vi "Subvi_Online_For_Offline_Analysis_For_Checking_LDAMatrix_w_weight.vi"(0 "rate":dbl=500.0 caption="Rate" format="%0.2f", 1 "samples per channel":i32=25, 5 "Brain_data_source":dbl[][](array[numeric]) caption="EEG_Raw_Data" format="%0.3f", 7 "Target_Flash_Order":i64[][](array[numeric]), 8 "Value":T1, 9 "사용할 Parameter 갯수":i32=2, 10 "Weight":dbl[](array[numeric]), 11 "Path":path, 14 "Number":string, 16 "Matrix":T1, 17 "Channel selection":bool[](array[boolean])) -> (13 "Array":dbl[](array[numeric]), 15 "자극별 ERP 발생여부":i16[](array[numeric]), 20 "output-0~8":i32, 24 "ERP_all":dbl[][](array[numeric]), 25 "자극별 ERP 발생 총 횟수":i16[](array[numeric]))   [LabVIEW 2014]
uses:
  <vilib>/Analysis/Matrix/Datatypes/RealMatrix.ctl
  <vilib>/Analysis/3filter.llb/Filter Passband Type.ctl
  <vilib>/Analysis/baseanly.llb/Real A x B.vi
  <vilib>/Analysis/baseanly.llb/Mean (DBL).vi
  <vilib>/Analysis/3filter.llb/Butterworth Filter (DBL).vi
  <vilib>/Analysis/Matrix/Numeric/Conversions/Array To Matrix - RA.vi
  <vilib>/Analysis/Matrix/Numeric/Conversions/Array To Matrix - RA2.vi
  <vilib>/Analysis/Matrix/Numeric/Conversions/Matrix To Array - RM.vi
  <vilib>/Analysis/Matrix/Numeric/Multiply/Multiply - RM,RM.vi
  <vilib>/Analysis/Matrix/Numeric/Subtract/Subtract - RM,RM.vi
  <vilib>/Analysis/NI_AALBase.lvlib
  <vilib>/Analysis/Matrix/NI_Matrix.lvlib
  <vilib>/Utility/file.llb/Read From Spreadsheet File (DBL).vi
panel:
  out "Array 2":dbl[](array[numeric])
  out "EPR_발생_total":i16[](array[numeric])
  in  "LDA":path=path "C:/Users/Administrator/Desktop/공공복지안전사업연구-노수진/파일럿20130902/LDA_Matrix_Value.xls"
  out "최대값":dbl
  out "#channel":i32
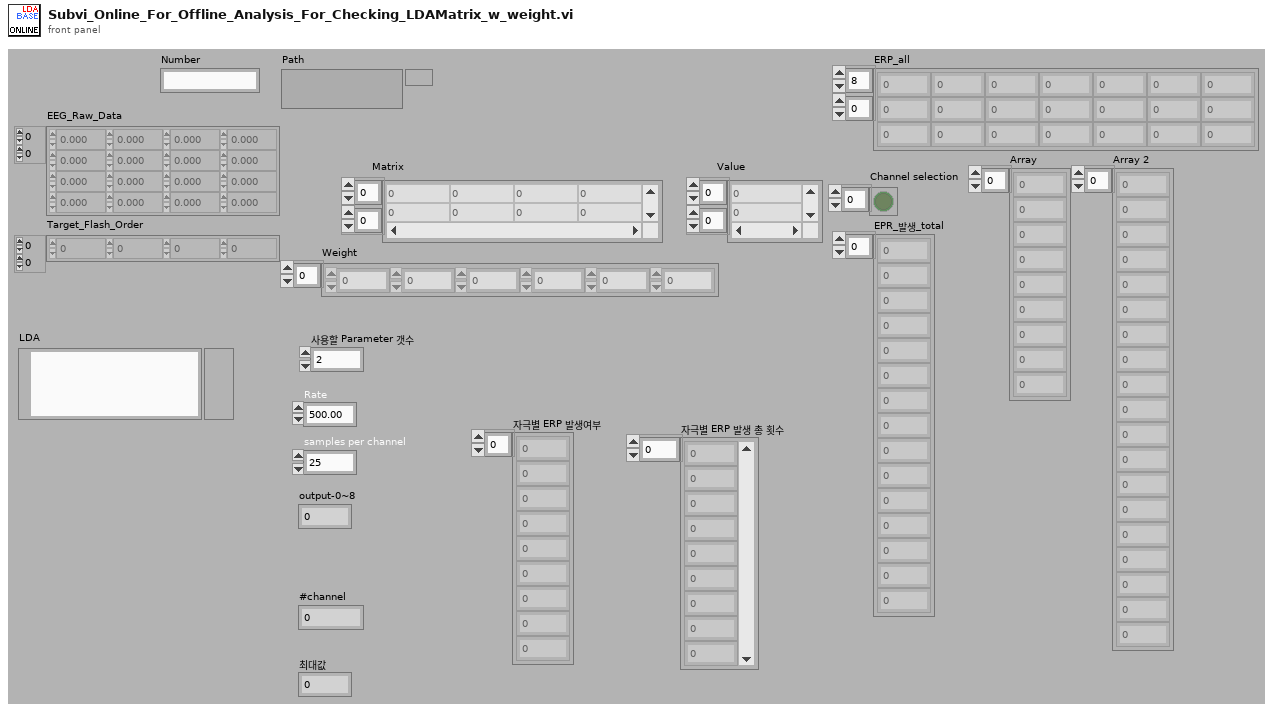
[diagram p1: front panel]
types:
  T1 = typedef "NI_Matrix.lvlib/RealMatrix.ctl" = dbl[][]
  T2 = typedef "NI_AALBase.lvlib/Filter Passband Type.ctl" = enum32{"Lowpass", "Highpass", "Bandpass", "Bandstop"}
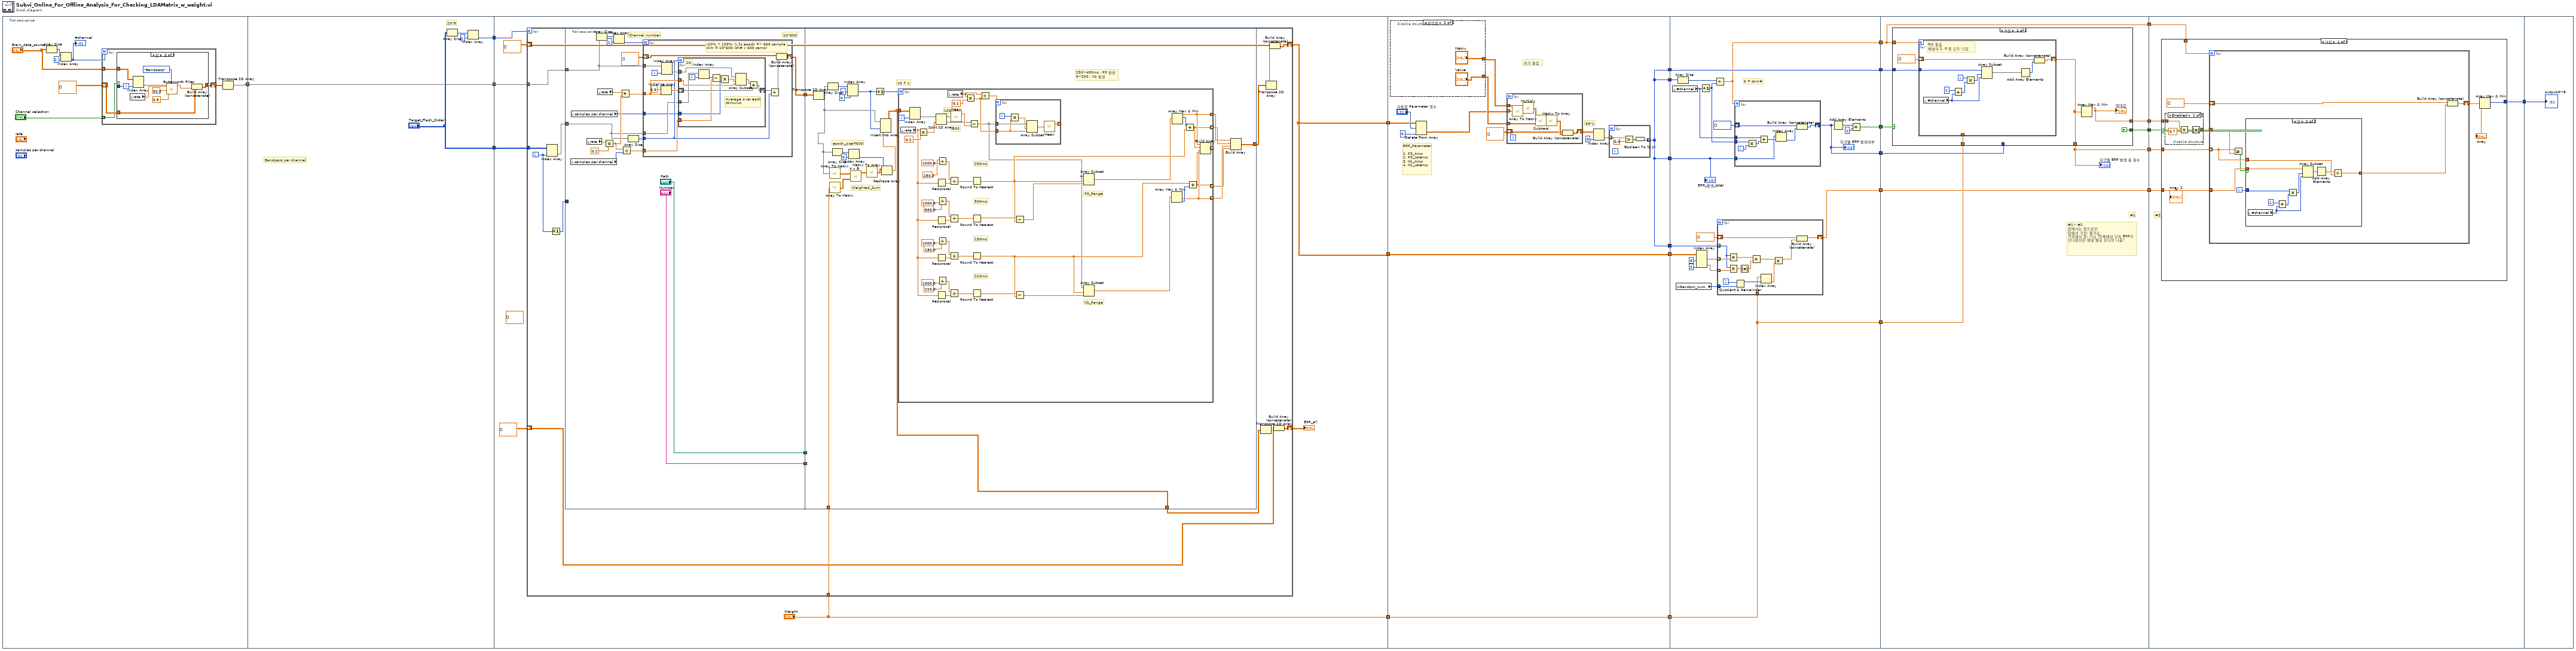
[diagram p0: block diagram]
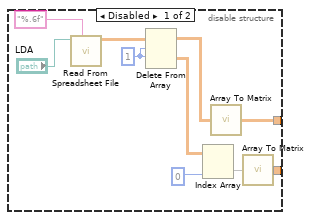
[diagram p3: hidden frame]
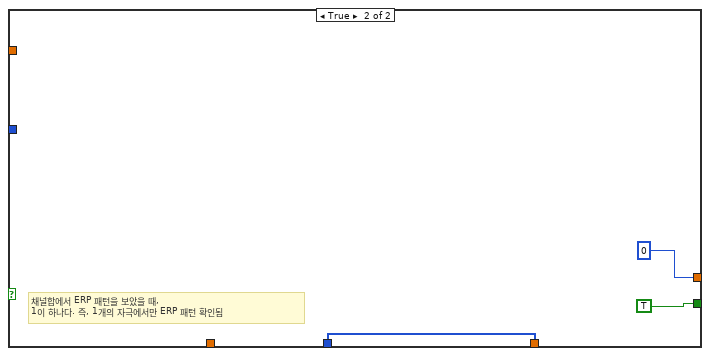
[diagram p4: hidden frame]
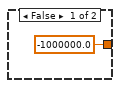
[diagram p6: hidden frame]
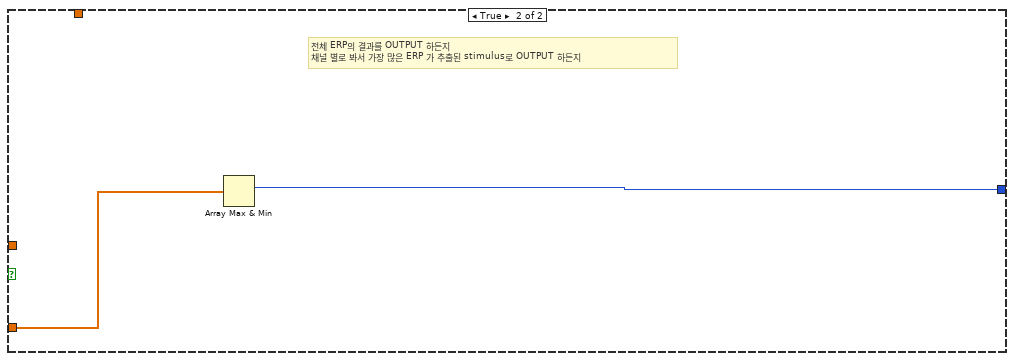
[diagram p7: hidden frame]
diagram:
  n1 = flat-sequence {
    tunnel: [w26] -> w25
    tunnel: [w50] -> w24
    tunnel: ["Target_Flash_Order"] -> w23
    tunnel: w25 -> [w50]
    tunnel: [w52] -> w22
    tunnel: w24 -> [w62]
    tunnel: w23 -> [w61]
    tunnel: w22 -> [w60]
    tunnel: [w55] -> w21
    tunnel: [w55] -> w20
    tunnel: ["Weight"] -> w3
    tunnel: w21 -> [w206]
    tunnel: [w202] -> w19
    tunnel: w20 -> [w202]
    tunnel: [w209] -> w17
    tunnel: [w209] -> w16
    tunnel: [w209] -> w15
    tunnel: [w209] -> w11
    tunnel: w3 -> [w201]
    tunnel: [w201] -> w2
    tunnel: w19 -> [w244]
    tunnel: [w250] -> w18
    tunnel: w17 -> [w250]
    tunnel: w16 -> [w260]
    tunnel: w15 -> [w257]
    tunnel: [w252] -> w14
    tunnel: [w251] -> w13
    tunnel: [w249] -> w12
    tunnel: w11 -> [w245]
    tunnel: [w243] -> w5
    tunnel: w2 -> [w239]
    tunnel: [w239] -> w1
    tunnel: w18 -> [w292]
    tunnel: w14 -> [w293]
    tunnel: w13 -> [w288]
    tunnel: w12 -> [w289]
    tunnel: [w291] -> w10
    tunnel: [w290] -> w9
    tunnel: [w289] -> w8
    tunnel: [w287] -> w6
    tunnel: w5 -> [w287]
    tunnel: [w286] -> w4
    tunnel: w1 -> [w285]
    tunnel: [w316] -> w7
    tunnel: w8 -> [w317]
    tunnel: w9 -> [w318]
    tunnel: w10 -> [w319]
    tunnel: w6 -> [w315]
    tunnel: w4 -> [w314]
    tunnel: w7 -> [w353]
    frame #0 {
      n2 = Array Size(array="Brain_data_source") -> (size(s)=w31:i32[])
      n3 = Index Array(array=w31, index=1) -> (element=w33:i32)
      "#channel" <- w33
      n4 = for {
        N: w33 -> [_]
        tunnel: "Brain_data_source" -> [w38]
        shift-right: [w35] -> w27
        shift-left: dbl[][] [] ("Filtered X") -> [w36]
        tunnel: "Channel selection" -> [w34] mode=indexing
        i -> [w37]
        n5 = case shown="참" w34 {
          tunnel: w38 -> [_ w49]
          tunnel: w37 -> [_ w48]
          tunnel: w36 -> [w39 w42]
          tunnel: [w39 w41] -> w35
          frame False {
          }
          frame True {
            n6 = local read "rate"() -> (w43:dbl)
            n7 = Index Array(array=w49, index (col)=w48) -> (element=w47:dbl[])  [unwired: 1 in]
            n8 = call-poly <vilib>:"Butterworth Filter.vi"("filter type"=Filter_Passband_Type."Bandpass", "low cutoff freq: fl"=0.5, "high cutoff freq: fh"=30.0, "sampling freq: fs"=w43, "X"=w47) -> ("Filtered X"=w40:dbl[])  [unwired: 3 in, 1 out]
            n9 = Build Array (concatenate)(w42, w40) -> (w41:dbl[][])
          }
        }
      }
      n10 = Transpose 2D Array(2D array=w27) -> (transposed array=w26:dbl[][])
    }
    frame #1 {
      # "Bandpass per channel"
      # "20*9"
      n11 = Array Size(array="Target_Flash_Order") -> (size(s)=w54:i32[])
      n12 = Index Array(array=w54, index=1 ("인덱스")) -> (element=w52:i32)
    }
    frame #2 {
      (unwired) dbl[][] []
      n13 = for {
        N: w60 -> [_]
        tunnel: w62 -> [w77]
        tunnel: w61 -> [w76]
        shift-right: [w73] -> w55
        shift-left: dbl[][] [] -> [w72]
        shift-right: [w67] -> w57
        shift-left: dbl[][] [] -> [w66]
        tunnel: "Weight" -> [w63]
        i -> [w71]
        n14 = Index Array(array=w76, index (col)=w71) -> (element=w75:i64[])  [unwired: 1 in]
        n15 = Increment(x=w71) -> (x+1=w70:i32)
        n16 = flat-sequence {
          tunnel: w77 -> [w84]
          tunnel: w75 -> [w83]
          tunnel: [w82] -> w79
          tunnel: w70 -> [_]
          tunnel: ["Path"] -> w69
          tunnel: ["Number"] -> w68
          tunnel: w79 -> [w143]
          tunnel: [w128] -> w78
          tunnel: w69 -> [_]
          tunnel: w68 -> [_]
          tunnel: [w130] -> w64
          tunnel: w63 -> [w132]
          frame #0 {
            # "10*600"
            # "Channel number"
            n17 = local read "samples per channel"() -> (w91:i32)
            n18 = local read "samples per channel"() -> (w90:i32)
            n19 = local read "rate"() -> (w93:dbl)
            n20 = Array Size(array=w84) -> (size(s)=w87:i32[])
            n21 = local read "rate"() -> (w95:dbl)
            n22 = Multiply(x=w93, y=0.2) -> (x*y=w97:dbl)
            n23 = Index Array(array=w87, index=1) -> (element=w89:i32)
            n24 = Add(x=w95, y=w97) -> (x+y=w96:dbl)
            n25 = Divide(x=w97, y=w91) -> (x/y=w94:dbl)
            n26 = Array Size(array=w83) -> (size(s)=w86:i32)
            n27 = for {
              N: w89 -> [_]
              tunnel: w90 -> [w98]
              tunnel: w96 -> [w109]
              shift-right: [w102] -> w82
              shift-left: dbl[][] [] -> [w104]
              tunnel: w86 -> [w103]
              tunnel: w84 -> [w101]
              tunnel: w83 -> [w100]
              tunnel: w94 -> [w99]
              i -> [w111]
              # "-20% ~ 100%: 1.2s epoch => 600 sample\ndim = 10*600 (ch# x 600 samp)"
              n28 = Initialize Array(0.0 ("element"), w109) -> (w108:dbl[])
              n29 = Index Array(array=w101, index (col)=w111) -> (element=w110:dbl[])  [unwired: 1 in]
              n30 = for {
                N: w103 -> [_]
                tunnel: w110 -> [w123]
                shift-right: [w120] -> w106
                shift-left: w108 -> [w121]
                tunnel: w109 -> [w119]
                tunnel: w100 -> [w117]
                tunnel: w99 -> [w115]
                tunnel: w98 -> [w113]
                i -> [w118]
                # "Average over each\nstimulus"
                # "20"
                n31 = Index Array(array=w117, index=w118) -> (element=w116:i64)
                n32 = Subtract(x=w116, y=w115) -> (x-y=w114:dbl)
                n33 = Multiply(x=w114, y=w113) -> (x*y=w112:dbl)
                n34 = Array Subset(array=w123, index=w112, length=w119) -> (w122:dbl[])
                n35 = Add(x=w122, y=w121) -> (x+y=w120:dbl[])
              }
              n36 = Divide(x=w106, y=w103) -> (x/y=w105:dbl[])
              n37 = Build Array (concatenate)(w104, w105) -> (w102:dbl[][])
            }
          }
          frame #1 {
            # "Weighted_Sum"
            # "epoch_size=600"
            # "250~450ms : P3 발생\n0~200 : N1 발생"
            # "10 + 1"
            n38 = Transpose 2D Array(2D array=w143) -> (transposed array=w129:dbl[][])
            n39 = Array Size(array=w129) -> (size(s)=w144:i32[])
            n40 = call-poly <vilib>:"Array To Matrix.vi"("Real 1D Array"=w132) -> ("Real Matrix (Column Vector)"=w138:T1)
            n41 = call-poly <vilib>:"Array To Matrix.vi"("Real 2D Array"=w129) -> ("Real Matrix"=w139:T1)
            n42 = Array Size(array=w129) -> (size(s)=w134:i32[])
            n43 = Index Array(array=w144, index #1=1 ("index"), index #2=0 ("인덱스")) -> (element #1=w140:i32)  [unwired: 1 out]
            n44 = Index Array(array=w134, index=0) -> (element=w133:i32)
            n45 = call-poly <vilib>:"A x B.vi"("B"=w138, "A"=w139) -> ("A x B"=w137:T1)  [unwired: 1 out]
            n46 = call-poly <vilib>:"Matrix To Array.vi"("Real Matrix"=w137) -> ("Real 2D Array"=w135:dbl[][])
            n47 = Increment(x=w140) -> (x+1=w141:i32)
            n48 = Reshape Array(w135, w133) -> (w131:dbl[])
            n49 = Insert Into Array(array=w129, index (col)=w140, new element=w131) -> (w130:dbl[][])  [unwired: 1 in]
            n50 = for {
              N: w141 -> [_]
              tunnel: w130 -> [w194]
              tunnel: [w150] -> w127 mode=indexing
              tunnel: [w149] -> w126 mode=indexing
              tunnel: [w148] -> w124 mode=indexing
              tunnel: [w147] -> w125 mode=indexing
              tunnel: [w146] -> _ mode=indexing
              i -> [w183]
              # "N1_Range"
              # "P3_Range"
              # "220ms"
              # "150ms"
              # "500ms"
              # "250ms"
              # "500"
              # "100"
              n51 = local read "rate"() -> (w164:dbl)
              n52 = Index Array(array=w194, index (col)=w183) -> (element=w185:dbl[])  [unwired: 1 in]
              n53 = Multiply(x=w164, y=0.2) -> (x*y=w192:dbl)
              n54 = Split 1D Array(array=w185, index=w192) -> (first subarray=w191:dbl[], second subarray=w182:dbl[])
              n55 = Reciprocal(x=w164) -> (1/x=w180:dbl)
              n56 = Reciprocal(x=w164) -> (1/x=w179:dbl)
              n57 = Reciprocal(x=w164) -> (1/x=w178:dbl)
              n58 = Reciprocal(x=w164) -> (1/x=w177:dbl)
              n59 = Divide(x=250.0, y=1000.0) -> (x/y=w176:dbl)
              n60 = Divide(x=500.0, y=1000.0) -> (x/y=w175:dbl)
              n61 = Divide(x=150.0, y=1000.0) -> (x/y=w174:dbl)
              n62 = Divide(x=220.0, y=1000.0) -> (x/y=w173:dbl)
              n63 = local read "rate"() -> (w188:dbl)
              n64 = Divide(x=w176, y=w180) -> (x/y=w163:dbl)
              n65 = Divide(x=w175, y=w179) -> (x/y=w162:dbl)
              n66 = Divide(x=w174, y=w178) -> (x/y=w161:dbl)
              n67 = Divide(x=w173, y=w177) -> (x/y=w160:dbl)
              n68 = call-poly <vilib>:"Mean.vi"("X"=w191) -> ("mean"=w190:dbl)  [unwired: 1 out]
              n69 = Multiply(x=w188, y=0.1) -> (x*y=w181:dbl)
              n70 = Subtract(x=w182, y=w190) -> (x-y=w151:dbl[])
              n71 = Round To Nearest(number=w163) -> (nearest integer value=w152:dbl)
              n72 = Round To Nearest(number=w162) -> (nearest integer value=w159:dbl)
              n73 = Round To Nearest(number=w161) -> (nearest integer value=w153:dbl)
              n74 = Round To Nearest(number=w160) -> (nearest integer value=w158:dbl)
              n75 = Divide(x=w188, y=w181) -> (x/y=w187:dbl)
              n76 = for {
                N: w187 -> [_]
                tunnel: w151 -> [w199]
                tunnel: [w200] -> _ mode=indexing
                tunnel: w181 -> [w197]
                i -> [w196]
                n77 = Multiply(x=w196, y=w197) -> (x*y=w198:dbl)
                n78 = Array Subset(array=w199, index=w198, length=w197) -> (w195:dbl[])
                n79 = call-poly <vilib>:"Mean.vi"("X"=w195) -> ("mean"=w200:dbl)  [unwired: 1 out]
              }
              n80 = Subtract(x=w159, y=w152) -> (x-y=w157:dbl)
              n81 = Subtract(x=w158, y=w153) -> (x-y=w156:dbl)
              n82 = Array Subset(array=w151, index=w152, length=w157) -> (w155:dbl[])
              n83 = Array Subset(array=w151, index=w153, length=w156) -> (w154:dbl[])
              n84 = Array Max & Min(array=w154) -> (min value=w148:dbl, min index (indices)=w184:i32)  [unwired: 2 out]
              n85 = Array Max & Min(array=w155) -> (max value=w150:dbl, max index (indices)=w186:i32)  [unwired: 2 out]
              n86 = Add(x=w186, y=w152) -> (x+y=w149:dbl)
              n87 = Add(x=w153, y=w184) -> (x+y=w147:dbl)
              n88 = Build Array(w150, w149, w148, w147) -> (w146:dbl[])
            }
            n89 = Build Array(w127, w126, w124, w125) -> (w128:dbl[][])
          }
        }
        n90 = Transpose 2D Array(2D array=w64) -> (transposed array=w65:dbl[][])
        n91 = Transpose 2D Array(2D array=w78) -> (transposed array=w74:dbl[][])
        n92 = Build Array (concatenate)(w72, w74) -> (w73:dbl[][])
        n93 = Build Array (concatenate)(w66, w65) -> (w67:dbl[][])
      }
      "ERP_all" <- w57
    }
    frame #3 {
      # "여기 틀림"
      # "ERP_Parameter\n\n1. P3_Amp\n2. P3_Latency\n3. N1_Amp\n4. N1_Latency"
      # "99*1"
      n94 = disable-structure shown="활성화" {
        disable-tunnel: [w218 "Matrix"] -> w208
        disable-tunnel: [w217 "Value"] -> w207
        frame Disabled {
          w220 = 1 ("인덱스 (행)")
          n95 = call-poly <vilib>:"Read From Spreadsheet File.vi"("format (%.3f)"="%.6f", "file path (dialog if empty)"="LDA") -> ("all rows"=w214:dbl[][])  [unwired: 5 in, 4 out]
          n96 = Delete From Array(array=w214, length=w220, index (row)=w220) -> (deleted portion=w223:dbl[][], array with subset deleted=w222:dbl[][])  [unwired: 1 in]
          n97 = Index Array(array=w223, index (col)=0 ("인덱스")) -> (element=w221:dbl[])  [unwired: 1 in]
          n98 = call-poly <vilib>:"Array To Matrix.vi"("Real 2D Array"=w222) -> ("Real Matrix"=w218:T1)
          n99 = call-poly <vilib>:"Array To Matrix.vi"("Real 1D Array"=w221) -> ("Real Matrix (Column Vector)"=w217:T1)
        }
        frame Enabled {
        }
      }
      n100 = Delete From Array(array=w206, length="사용할 Parameter 갯수", index (col)=0 ("비활성화된 인덱스 (열)")) -> (deleted portion=w204:dbl[][])  [unwired: 1 in, 1 out]
      n101 = for {
        tunnel: w208 -> [w238]
        tunnel: w207 -> [w235]
        shift-right: [w232] -> w210
        shift-left: dbl[][] [] -> [w231]
        tunnel: w204 -> [w230] mode=indexing
        n102 = call-poly <vilib>:"Array To Matrix.vi"("Real 1D Array"=w230) -> ("Real Matrix (Column Vector)"=w234:T1)
        n103 = call-poly <vilib>:"Multiply.vi"("Real Matrix B"=w234, "Real Matrix A"=w238) -> ("A * B"=w237:T1)
        n104 = call-poly <vilib>:"Subtract.vi"("Real Matrix B"=w235, "Real Matrix A"=w237) -> ("A - B"=w236:T1)
        n105 = call-poly <vilib>:"Matrix To Array.vi"("Real Matrix"=w236) -> ("Real 2D Array"=w233:dbl[][])
        n106 = Build Array (concatenate)(w231, w233) -> (w232:dbl[][])
      }
      n107 = Index Array(array=w210, index (col)=0 ("비활성화된 인덱스 (열)")) -> (element=w211:dbl[])  [unwired: 1 in]
      n108 = for {
        tunnel: w211 -> [w229] mode=indexing
        tunnel: [w228] -> w209 mode=indexing
        n109 = Greater?(x=w229, y=0.0) -> (0:w226:bool)
        n110 = Boolean To (0,1)(Boolean=w226) -> (0, 1=w228:i16)
      }
    }
    frame #4 {
      # "6 = stim#"
      n111 = local read "#channel"() -> (w255:i32)
      n112 = global read "Control_Panel_정리.vi" "Random_num"() -> (w240:i32)
      n113 = Array Size(array=w260) -> (size(s)=w259:i32)
      n114 = Index Array(array=w244, index (col) #1=0 ("비활성화된 인덱스 (열)"), index (col) #2=2 ("인덱스 (열)")) -> (element #1=w247:dbl[], element #2=w241:dbl[])  [unwired: 2 in]
      n115 = Increment(x=w255) -> (x+1=w258:i32)
      n116 = Divide(x=w259, y=w258) -> (x/y=w249:dbl)
      n117 = for {
        tunnel: w245 -> [w272] mode=indexing
        tunnel: w247 -> [w275] mode=indexing
        shift-right: [w273] -> w243
        shift-left: dbl[] [] -> [w274]
        tunnel: w241 -> [w271] mode=indexing
        tunnel: w240 -> [w265]
        tunnel: w239 -> [w261]
        i -> [w266]
        n118 = Multiply(x=w272, y=w275) -> (x*y=w269:dbl)
        n119 = Multiply(x=w272, y=w271) -> (x*y=w267:dbl)
        n120 = Quotient & Remainder(x=w266, y=w265) -> (x-y*floor(x/y)=w264:i32)  [unwired: 1 out]
        n121 = Absolute Value(x=w267) -> (abs(x)=w270:dbl)
        n122 = Add(x=w269, y=w270) -> (x+y=w268:dbl)
        n123 = Index Array(array=w261, index=w264) -> (element=w262:dbl)
        n124 = Multiply(x=w268, y=w262) -> (x*y=w263:dbl)
        n125 = Build Array (concatenate)(w274, w263) -> (w273:dbl[])
      }
      n126 = for {
        N: w249 -> [_]
        tunnel: w258 -> [w283]
        tunnel: w255 -> [w281]
        tunnel: w257 -> [w280]
        shift-right: [w277] -> w251
        shift-left: i16[] [] -> [w278]
        i -> [w284]
        n127 = Multiply(x=w283, y=w284) -> (x*y=w282:i32)
        n128 = Add(x=w281, y=w282) -> (x+y=w276:i32)
        n129 = Index Array(array=w280, index=w276) -> (element=w279:i16)
        n130 = Build Array (concatenate)(w278, w279) -> (w277:i16[])
      }
      "자극별 ERP 발생여부" <- w251
      n131 = Add Array Elements(numeric array=w251) -> (sum=w254:i16)
      n132 = Equal?(x=w254, y=i16 1) -> (x = y?=w252:bool)
      "EPR_발생_total" <- w257
    }
    frame #5 {
      # "#1> #2\n참에서는 참으로만\n참에서 거짓: 불가능\n거짓에서 참: 가능 (전체에선 단독 ERP가 안나왔지만 채널 별로 보니까 나옴)"
      # "#1"
      n133 = case shown="거짓" w293 {
        tunnel: w292 -> [w300 _]
        tunnel: w289 -> [w299 _]
        tunnel: [FALSE TRUE] -> w291
        tunnel: [w298 0] -> w290
        tunnel: w288 -> [_ w311]
        tunnel: [w297 w311] -> w286
        tunnel: w285 -> [w295 _]
        frame False {
          n134 = for {
            N: w299 -> [_]
            tunnel: w300 -> [w310]
            shift-right: [w302] -> w297
            shift-left: dbl[] [] -> [w303]
            tunnel: w295 -> [_]
            i -> [w309]
            # "9번 돌음\n채널의 1, 0 을 모두 더함"
            n135 = local read "#channel"() -> (w308:i32)
            n136 = Add(x=1, y=w308) -> (x+y=w306:i32)
            n137 = Multiply(x=w309, y=w306) -> (x*y=w305:i32)
            n138 = Array Subset(array=w310, index=w305, length=w308) -> (w301:i16[])
            n139 = Add Array Elements(numeric array=w301) -> (sum=w304:i16)
            n140 = Build Array (concatenate)(w303, w304) -> (w302:dbl[])
          }
          n141 = Array Max & Min(array=w297) -> (max value=w298:dbl)  [unwired: 3 out]
          "최대값" <- w298
        }
        frame True {
          # "채널합에서 ERP 패턴을 보았을 때,\n1이 하나다. 즉, 1개의 자극에서만 ERP 패턴 확인됨"
        }
      }
      "자극별 ERP 발생 총 횟수" <- w286
    }
    frame #6 {
      # "#2"
      n142 = case shown="거짓" w319 {
        tunnel: w318 -> [w322 _]
        tunnel: w317 -> [w327 _]
        tunnel: [w323 w352] -> w316
        tunnel: w315 -> [w326 _]
        tunnel: w314 -> [w325 w351]
        frame False {
          n143 = disable-structure shown="Enabled" {
            disable-tunnel: w322 -> [w331 _]
            disable-tunnel: [w328 _] -> w321
            frame Enabled {
              n144 = Multiply(x=w331, y=0.7) -> (x*y=w329:dbl)
              n145 = Absolute Value(x=w329) -> (abs(x)=w328:dbl)
            }
            frame Disabled {
            }
          }
          n146 = for {
            N: w327 -> [_]
            tunnel: w326 -> [w334]
            tunnel: w325 -> [w335] mode=indexing
            shift-right: [w336] -> w320
            shift-left: dbl[] [] -> [w337]
            tunnel: w321 -> [w333]
            i -> [w339]
            n147 = Greater Or Equal?(x=w335, y=w333) -> (x >= y?=w332:bool)
            n148 = case shown="참" w332 {
              tunnel: w339 -> [_ w350]
              tunnel: [-1000000.0 w349] -> w338
              tunnel: w335 -> [_ w348]
              tunnel: w334 -> [_ w347]
              frame False {
              }
              frame True {
                n149 = local read "#channel"() -> (w343:i32)
                n150 = Add(x=1, y=w343) -> (x+y=w345:i32)
                n151 = Multiply(x=w350, y=w345) -> (x*y=w344:i32)
                n152 = Array Subset(array=w347, index=w344, length=w343) -> (w342:dbl[])
                n153 = Add Array Elements(numeric array=w342) -> (sum=w341:dbl)
                n154 = Divide(x=w341, y=w348) -> (x/y=w349:dbl)
              }
            }
            n155 = Build Array (concatenate)(w337, w338) -> (w336:dbl[])
          }
          "Array" <- w320
          n156 = Array Max & Min(array=w320) -> (max index (indices)=w323:i32)  [unwired: 3 out]
          "Array 2" <- w326
        }
        frame True {
          # "전체 ERP의 결과를 OUTPUT 하든지\n채널 별로 봐서 가장 많은 ERP 가 추출된 stimulus로 OUTPUT 하든지"
          n157 = Array Max & Min(array=w351) -> (max index (indices)=w352:i32)  [unwired: 3 out]
        }
      }
    }
    frame #7 {
      "output-0~8" <- w353
    }
  }
